vi "File.Create Folder if Does Not Exist.vi"(8 "error in":errorcluster, 11 "Path":path) -> (0 "error out":errorcluster, 2 "Created":bool, 3 "Dup Path":path)   [LabVIEW 2024, in "EQMF.lvlib" / "File Utils.lvlib"]
uses:
  File Utils.lvlib
  Status/Status Utils.lvlib
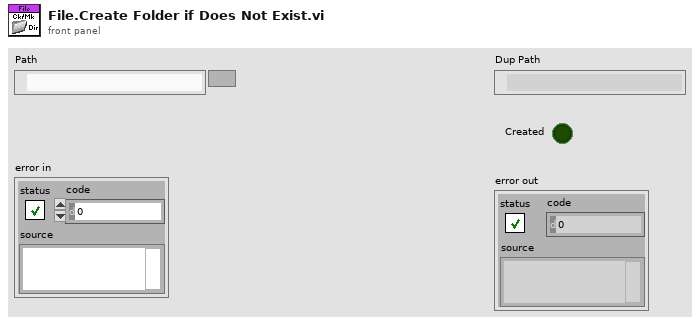
[diagram p1: front panel]
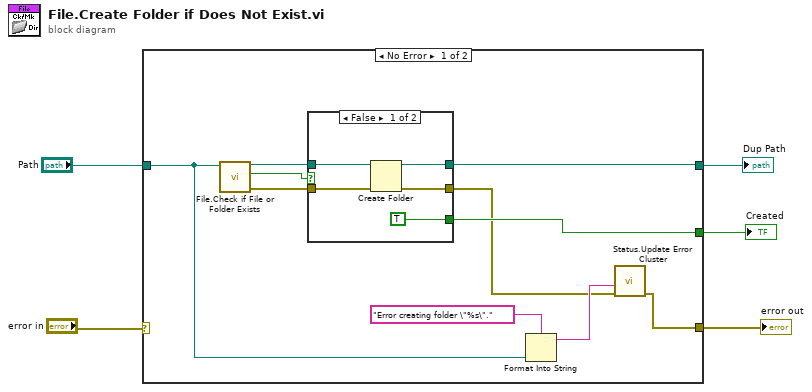
[diagram p0: block diagram]
diagram:
  n1 = case shown="No Error" "error in" {
    selector: "error in" -> [_ w24]
    tunnel: "Path" -> [w8 w23]
    tunnel: [w11 _] -> w4
    tunnel: [w6 w24] -> w2
    tunnel: [w13 w23] -> w1
    frame No Error {
      n2 = call "File.Check if File or Folder Exists.vi"("Path"=w8) -> ("error out"=w14:errorcluster, "Exists"=w12:bool, "Dup Path"=w15:path)  [unwired: 6 in, 2 out]
      n3 = case shown="False" w12 {
        tunnel: w15 -> [w20 w22]
        tunnel: w14 -> [w19 w21]
        tunnel: [w18 w21] -> w7
        tunnel: [w17 w22] -> w13
        tunnel: [TRUE _] -> w11
        frame False {
          n4 = Create Folder(path (use dialog)=w20, error in=w19) -> (created path=w17:path, error out=w18:errorcluster)  [unwired: 1 in, 1 out]
        }
        frame True {
        }
      }
      n5 = Format Into String(format string="Error creating folder \"%s\".", w8) -> (resulting string=w10:string)  [unwired: 2 in, 1 out]
      n6 = call "Status.Update Error Cluster.vi"("Error In"=w7, "NewDesc"=w10) -> ("Error Out"=w6:errorcluster)  [unwired: 9 in]
    }
    frame Error {
    }
  }
  "Created" <- w4
  "error out" <- w2
  "Dup Path" <- w1
